vi "FipsAdjacent.vi"() -> (11 "Fips":i32[](array[numeric]))   [LabVIEW 2017] (continued)
WA\"\t53075\t\"Nez Perce County, ID\"\t16069\n\"Whitman County, WA\"\t53075\t\"Adams County, WA\"\t53001\n\"Whitman County, WA\"\t53075\t\"Asotin County, WA\"\t53003\n\"Whitman County, WA\"\t53075\t\"Columbia County, WA\"\t53013\n\"Whitman County, WA\"\t53075\t\"Franklin County, WA\"\t53021\n\"Whitman County, WA\"\t53075\t\"Garfield County, WA\"\t53023\n\"Whitman County, WA\"\t53075\t\"Lincoln County, WA\"\t53043\n\"Whitman County, WA\"\t53075\t\"Spokane County, WA\"\t53063\n\"Whitman County, WA\"\t53075\t\"Whitman County, WA\"\t53075\n\"Yakima County, WA\"\t53077\t\"Benton County, WA\"\t53005\n\"Yakima County, WA\"\t53077\t\"Grant County, WA\"\t53025\n\"Yakima County, WA\"\t53077\t\"King County, WA\"\t53033\n\"Yakima County, WA\"\t53077\t\"Kittitas County, WA\"\t53037\n\"Yakima County, WA\"\t53077\t\"Klickitat County, WA\"\t53039\n\"Yakima County, WA\"\t53077\t\"Lewis County, WA\"\t53041\n\"Yakima County, WA\"\t53077\t\"Pierce County, WA\"\t53053\n\"Yakima County, WA\"\t53077\t\"Skamania County, WA\"\t53059\n\"Yakima County, WA\"\t53077\t\"Yakima County, WA\"\t53077\n\"Barbour County, WV\"\t54001\t\"Barbour County, WV\"\t54001\n\"Barbour County, WV\"\t54001\t\"Harrison County, WV\"\t54033\n\"Barbour County, WV\"\t54001\t\"Preston County, WV\"\t54077\n\"Barbour County, WV\"\t54001\t\"Randolph County, WV\"\t54083\n\"Barbour County, WV\"\t54001\t\"Taylor County, WV\"\t54091\n\"Barbour County, WV\"\t54001\t\"Tucker County, WV\"\t54093\n\"Barbour County, WV\"\t54001\t\"Upshur County, WV\"\t54097\n\"Berkeley County, WV\"\t54003\t\"Washington County, MD\"\t24043\n\"Berkeley County, WV\"\t54003\t\"Clarke County, VA\"\t51043\n\"Berkeley County, WV\"\t54003\t\"Frederick County, VA\"\t51069\n\"Berkeley County, WV\"\t54003\t\"Berkeley County, WV\"\t54003\n\"Berkeley County, WV\"\t54003\t\"Jefferson County, WV\"\t54037\n\"Berkeley County, WV\"\t54003\t\"Morgan County, WV\"\t54065\n\"Boone County, WV\"\t54005\t\"Boone County, WV\"\t54005\n\"Boone County, WV\"\t54005\t\"Kanawha County, WV\"\t54039\n\"Boone County, WV\"\t54005\t\"Lincoln County, WV\"\t54043\n\"Boone County, WV\"\t54005\t\"Logan County, WV\"\t54045\n\"Boone County, WV\"\t54005\t\"Raleigh County, WV\"\t54081\n\"Boone County, WV\"\t54005\t\"Wyoming County, WV\"\t54109\n\"Braxton County, WV\"\t54007\t\"Braxton County, WV\"\t54007\n\"Braxton County, WV\"\t54007\t\"Calhoun County, WV\"\t54013\n\"Braxton County, WV\"\t54007\t\"Clay County, WV\"\t54015\n\"Braxton County, WV\"\t54007\t\"Gilmer County, WV\"\t54021\n\"Braxton County, WV\"\t54007\t\"Lewis County, WV\"\t54041\n\"Braxton County, WV\"\t54007\t\"Nicholas County, WV\"\t54067\n\"Braxton County, WV\"\t54007\t\"Webster County, WV\"\t54101\n\"Brooke County, WV\"\t54009\t\"Jefferson County, OH\"\t39081\n\"Brooke County, WV\"\t54009\t\"Washington County, PA\"\t42125\n\"Brooke County, WV\"\t54009\t\"Brooke County, WV\"\t54009\n\"Brooke County, WV\"\t54009\t\"Hancock County, WV\"\t54029\n\"Brooke County, WV\"\t54009\t\"Ohio County, WV\"\t54069\n\"Cabell County, WV\"\t54011\t\"Gallia County, OH\"\t39053\n\"Cabell County, WV\"\t54011\t\"Lawrence County, OH\"\t39087\n\"Cabell County, WV\"\t54011\t\"Cabell County, WV\"\t54011\n\"Cabell County, WV\"\t54011\t\"Lincoln County, WV\"\t54043\n\"Cabell County, WV\"\t54011\t\"Mason County, WV\"\t54053\n\"Cabell County, WV\"\t54011\t\"Putnam County, WV\"\t54079\n\"Cabell County, WV\"\t54011\t\"Wayne County, WV\"\t54099\n\"Calhoun County, WV\"\t54013\t\"Braxton County, WV\"\t54007\n\"Calhoun County, WV\"\t54013\t\"Calhoun County, WV\"\t54013\n\"Calhoun County, WV\"\t54013\t\"Clay County, WV\"\t54015\n\"Calhoun County, WV\"\t54013\t\"Gilmer County, WV\"\t54021\n\"Calhoun County, WV\"\t54013\t\"Ritchie County, WV\"\t54085\n\"Calhoun County, WV\"\t54013\t\"Roane County, WV\"\t54087\n\"Calhoun County, WV\"\t54013\t\"Wirt County, WV\"\t54105\n\"Clay County, WV\"\t54015\t\"Braxton County, WV\"\t54007\n\"Clay County, WV\"\t54015\t\"Calhoun County, WV\"\t54013\n\"Clay County, WV\"\t54015\t\"Clay County, WV\"\t54015\n\"Clay County, WV\"\t54015\t\"Kanawha County, WV\"\t54039\n\"Clay County, WV\"\t54015\t\"Nicholas County, WV\"\t54067\n\"Clay County, WV\"\t54015\t\"Roane County, WV\"\t54087\n\"Doddridge County, WV\"\t54017\t\"Doddridge County, WV\"\t54017\n\"Doddridge County, WV\"\t54017\t\"Gilmer County, WV\"\t54021\n\"Doddridge County, WV\"\t54017\t\"Harrison County, WV\"\t54033\n\"Doddridge County, WV\"\t54017\t\"Lewis County, WV\"\t54041\n\"Doddridge County, WV\"\t54017\t\"Ritchie County, WV\"\t54085\n\"Doddridge County, WV\"\t54017\t\"Tyler County, WV\"\t54095\n\"Doddridge County, WV\"\t54017\t\"Wetzel County, WV\"\t54103\n\"Fayette County, WV\"\t54019\t\"Fayette County, WV\"\t54019\n\"Fayette County, WV\"\t54019\t\"Greenbrier County, WV\"\t54025\n\"Fayette County, WV\"\t54019\t\"Kanawha County, WV\"\t54039\n\"Fayette County, WV\"\t54019\t\"Nicholas County, WV\"\t54067\n\"Fayette County, WV\"\t54019\t\"Raleigh County, WV\"\t54081\n\"Fayette County, WV\"\t54019\t\"Summers County, WV\"\t54089\n\"Gilmer County, WV\"\t54021\t\"Braxton County, WV\"\t54007\n\"Gilmer County, WV\"\t54021\t\"Calhoun County, WV\"\t54013\n\"Gilmer County, WV\"\t54021\t\"Doddridge County, WV\"\t54017\n\"Gilmer County, WV\"\t54021\t\"Gilmer County, WV\"\t54021\n\"Gilmer County, WV\"\t54021\t\"Lewis County, WV\"\t54041\n\"Gilmer County, WV\"\t54021\t\"Ritchie County, WV\"\t54085\n\"Grant County, WV\"\t54023\t\"Garrett County, MD\"\t24023\n\"Grant County, WV\"\t54023\t\"Grant County, WV\"\t54023\n\"Grant County, WV\"\t54023\t\"Hampshire County, WV\"\t54027\n\"Grant County, WV\"\t54023\t\"Hardy County, WV\"\t54031\n\"Grant County, WV\"\t54023\t\"Mineral County, WV\"\t54057\n\"Grant County, WV\"\t54023\t\"Pendleton County, WV\"\t54071\n\"Grant County, WV\"\t54023\t\"Preston County, WV\"\t54077\n\"Grant County, WV\"\t54023\t\"Randolph County, WV\"\t54083\n\"Grant County, WV\"\t54023\t\"Tucker County, WV\"\t54093\n\"Greenbrier County, WV\"\t54025\t\"Alleghany County, VA\"\t51005\n\"Greenbrier County, WV\"\t54025\t\"Bath County, VA\"\t51017\n\"Greenbrier County, WV\"\t54025\t\"Fayette County, WV\"\t54019\n\"Greenbrier County, WV\"\t54025\t\"Greenbrier County, WV\"\t54025\n\"Greenbrier County, WV\"\t54025\t\"Monroe County, WV\"\t54063\n\"Greenbrier County, WV\"\t54025\t\"Nicholas County, WV\"\t54067\n\"Greenbrier County, WV\"\t54025\t\"Pocahontas County, WV\"\t54075\n\"Greenbrier County, WV\"\t54025\t\"Summers County, WV\"\t54089\n\"Greenbrier County, WV\"\t54025\t\"Webster County, WV\"\t54101\n\"Hampshire County, WV\"\t54027\t\"Allegany County, MD\"\t24001\n\"Hampshire County, WV\"\t54027\t\"Frederick County, VA\"\t51069\n\"Hampshire County, WV\"\t54027\t\"Grant County, WV\"\t54023\n\"Hampshire County, WV\"\t54027\t\"Hampshire County, WV\"\t54027\n\"Hampshire County, WV\"\t54027\t\"Hardy County, WV\"\t54031\n\"Hampshire County, WV\"\t54027\t\"Mineral County, WV\"\t54057\n\"Hampshire County, WV\"\t54027\t\"Morgan County, WV\"\t54065\n\"Hancock County, WV\"\t54029\t\"Columbiana County, OH\"\t39029\n\"Hancock County, WV\"\t54029\t\"Jefferson County, OH\"\t39081\n\"Hancock County, WV\"\t54029\t\"Beaver County, PA\"\t42007\n\"Hancock County, WV\"\t54029\t\"Washington County, PA\"\t42125\n\"Hancock County, WV\"\t54029\t\"Brooke County, WV\"\t54009\n\"Hancock County, WV\"\t54029\t\"Hancock County, WV\"\t54029\n\"Hardy County, WV\"\t54031\t\"Frederick County, VA\"\t51069\n\"Hardy County, WV\"\t54031\t\"Rockingham County, VA\"\t51165\n\"Hardy County, WV\"\t54031\t\"Shenandoah County, VA\"\t51171\n\"Hardy County, WV\"\t54031\t\"Grant County, WV\"\t54023\n\"Hardy County, WV\"\t54031\t\"Hampshire County, WV\"\t54027\n\"Hardy County, WV\"\t54031\t\"Hardy County, WV\"\t54031\n\"Hardy County, WV\"\t54031\t\"Mineral County, WV\"\t54057\n\"Hardy County, WV\"\t54031\t\"Pendleton County, WV\"\t54071\n\"Harrison County, WV\"\t54033\t\"Barbour County, WV\"\t54001\n\"Harrison County, WV\"\t54033\t\"Doddridge County, WV\"\t54017\n\"Harrison County, WV\"\t54033\t\"Harrison County, WV\"\t54033\n\"Harrison County, WV\"\t54033\t\"Lewis County, WV\"\t54041\n\"Harrison County, WV\"\t54033\t\"Marion County, WV\"\t54049\n\"Harrison County, WV\"\t54033\t\"Taylor County, WV\"\t54091\n\"Harrison County, WV\"\t54033\t\"Upshur County, WV\"\t54097\n\"Harrison County, WV\"\t54033\t\"Wetzel County, WV\"\t54103\n\"Jackson County, WV\"\t54035\t\"Meigs County, OH\"\t39105\n\"Jackson County, WV\"\t54035\t\"Jackson County, WV\"\t54035\n\"Jackson County, WV\"\t54035\t\"Kanawha County, WV\"\t54039\n\"Jackson County, WV\"\t54035\t\"Mason County, WV\"\t54053\n\"Jackson County, WV\"\t54035\t\"Putnam County, WV\"\t54079\n\"Jackson County, WV\"\t54035\t\"Roane County, WV\"\t54087\n\"Jackson County, WV\"\t54035\t\"Wirt County, WV\"\t54105\n\"Jackson County, WV\"\t54035\t\"Wood County, WV\"\t54107\n\"Jefferson County, WV\"\t54037\t\"Washington County, MD\"\t24043\n\"Jefferson County, WV\"\t54037\t\"Clarke County, VA\"\t51043\n\"Jefferson County, WV\"\t54037\t\"Frederick County, VA\"\t51069\n\"Jefferson County, WV\"\t54037\t\"Loudoun County, VA\"\t51107\n\"Jefferson County, WV\"\t54037\t\"Berkeley County, WV\"\t54003\n\"Jefferson County, WV\"\t54037\t\"Jefferson County, WV\"\t54037\n\"Kanawha County, WV\"\t54039\t\"Boone County, WV\"\t54005\n\"Kanawha County, WV\"\t54039\t\"Clay County, WV\"\t54015\n\"Kanawha County, WV\"\t54039\t\"Fayette County, WV\"\t54019\n\"Kanawha County, WV\"\t54039\t\"Jackson County, WV\"\t54035\n\"Kanawha County, WV\"\t54039\t\"Kanawha County, WV\"\t54039\n\"Kanawha County, WV\"\t54039\t\"Lincoln County, WV\"\t54043\n\"Kanawha County, WV\"\t54039\t\"Nicholas County, WV\"\t54067\n\"Kanawha County, WV\"\t54039\t\"Putnam County, WV\"\t54079\n\"Kanawha County, WV\"\t54039\t\"Raleigh County, WV\"\t54081\n\"Kanawha County, WV\"\t54039\t\"Roane County, WV\"\t54087\n\"Lewis County, WV\"\t54041\t\"Braxton County, WV\"\t54007\n\"Lewis County, WV\"\t54041\t\"Doddridge County, WV\"\t54017\n\"Lewis County, WV\"\t54041\t\"Gilmer County, WV\"\t54021\n\"Lewis County, WV\"\t54041\t\"Harrison County, WV\"\t54033\n\"Lewis County, WV\"\t54041\t\"Lewis County, WV\"\t54041\n\"Lewis County, WV\"\t54041\t\"Upshur County, WV\"\t54097\n\"Lewis County, WV\"\t54041\t\"Webster County, WV\"\t54101\n\"Lincoln County, WV\"\t54043\t\"Boone County, WV\"\t54005\n\"Lincoln County, WV\"\t54043\t\"Cabell County, WV\"\t54011\n\"Lincoln County, WV\"\t54043\t\"Kanawha County, WV\"\t54039\n\"Lincoln County, WV\"\t54043\t\"Lincoln County, WV\"\t54043\n\"Lincoln County, WV\"\t54043\t\"Logan County, WV\"\t54045\n\"Lincoln County, WV\"\t54043\t\"Mingo County, WV\"\t54059\n\"Lincoln County, WV\"\t54043\t\"Putnam County, WV\"\t54079\n\"Lincoln County, WV\"\t54043\t\"Wayne County, WV\"\t54099\n\"Logan County, WV\"\t54045\t\"Boone County, WV\"\t54005\n\"Logan County, WV\"\t54045\t\"Lincoln County, WV\"\t54043\n\"Logan County, WV\"\t54045\t\"Logan County, WV\"\t54045\n\"Logan County, WV\"\t54045\t\"Mingo County, WV\"\t54059\n\"Logan County, WV\"\t54045\t\"Wyoming County, WV\"\t54109\n\"McDowell County, WV\"\t54047\t\"Buchanan County, VA\"\t51027\n\"McDowell County, WV\"\t54047\t\"Tazewell County, VA\"\t51185\n\"McDowell County, WV\"\t54047\t\"McDowell County, WV\"\t54047\n\"McDowell County, WV\"\t54047\t\"Mercer County, WV\"\t54055\n\"McDowell County, WV\"\t54047\t\"Mingo County, WV\"\t54059\n\"McDowell County, WV\"\t54047\t\"Wyoming County, WV\"\t54109\n\"Marion County, WV\"\t54049\t\"Harrison County, WV\"\t54033\n\"Marion County, WV\"\t54049\t\"Marion County, WV\"\t54049\n\"Marion County, WV\"\t54049\t\"Monongalia County, WV\"\t54061\n\"Marion County, WV\"\t54049\t\"Taylor County, WV\"\t54091\n\"Marion County, WV\"\t54049\t\"Wetzel County, WV\"\t54103\n\"Marshall County, WV\"\t54051\t\"Belmont County, OH\"\t39013\n\"Marshall County, WV\"\t54051\t\"Monroe County, OH\"\t39111\n\"Marshall County, WV\"\t54051\t\"Greene County, PA\"\t42059\n\"Marshall County, WV\"\t54051\t\"Washington County, PA\"\t42125\n\"Marshall County, WV\"\t54051\t\"Marshall County, WV\"\t54051\n\"Marshall County, WV\"\t54051\t\"Ohio County, WV\"\t54069\n\"Marshall County, WV\"\t54051\t\"Wetzel County, WV\"\t54103\n\"Mason County, WV\"\t54053\t\"Gallia County, OH\"\t39053\n\"Mason County, WV\"\t54053\t\"Meigs County, OH\"\t39105\n\"Mason County, WV\"\t54053\t\"Cabell County, WV\"\t54011\n\"Mason County, WV\"\t54053\t\"Jackson County, WV\"\t54035\n\"Mason County, WV\"\t54053\t\"Mason County, WV\"\t54053\n\"Mason County, WV\"\t54053\t\"Putnam County, WV\"\t54079\n\"Mercer County, WV\"\t54055\t\"Bland County, VA\"\t51021\n\"Mercer County, WV\"\t54055\t\"Giles County, VA\"\t51071\n\"Mercer County, WV\"\t54055\t\"Tazewell County, VA\"\t51185\n\"Mercer County, WV\"\t54055\t\"McDowell County, WV\"\t54047\n\"Mercer County, WV\"\t54055\t\"Mercer County, WV\"\t54055\n\"Mercer County, WV\"\t54055\t\"Raleigh County, WV\"\t54081\n\"Mercer County, WV\"\t54055\t\"Summers County, WV\"\t54089\n\"Mercer County, WV\"\t54055\t\"Wyoming County, WV\"\t54109\n\"Mineral County, WV\"\t54057\t\"Allegany County, MD\"\t24001\n\"Mineral County, WV\"\t54057\t\"Garrett County, MD\"\t24023\n\"Mineral County, WV\"\t54057\t\"Grant County, WV\"\t54023\n\"Mineral County, WV\"\t54057\t\"Hampshire County, WV\"\t54027\n\"Mineral County, WV\"\t54057\t\"Hardy County, WV\"\t54031\n\"Mineral County, WV\"\t54057\t\"Mineral County, WV\"\t54057\n\"Mingo County, WV\"\t54059\t\"Martin County, KY\"\t21159\n\"Mingo County, WV\"\t54059\t\"Pike County, KY\"\t21195\n\"Mingo County, WV\"\t54059\t\"Buchanan County, VA\"\t51027\n\"Mingo County, WV\"\t54059\t\"Lincoln County, WV\"\t54043\n\"Mingo County, WV\"\t54059\t\"Logan County, WV\"\t54045\n\"Mingo County, WV\"\t54059\t\"McDowell County, WV\"\t54047\n\"Mingo County, WV\"\t54059\t\"Mingo County, WV\"\t54059\n\"Mingo County, WV\"\t54059\t\"Wayne County, WV\"\t54099\n\"Mingo County, WV\"\t54059\t\"Wyoming County, WV\"\t54109\n\"Monongalia County, WV\"\t54061\t\"Fayette County, PA\"\t42051\n\"Monongalia County, WV\"\t54061\t\"Greene County, PA\"\t42059\n\"Monongalia County, WV\"\t54061\t\"Marion County, WV\"\t54049\n\"Monongalia County, WV\"\t54061\t\"Monongalia County, WV\"\t54061\n\"Monongalia County, WV\"\t54061\t\"Preston County, WV\"\t54077\n\"Monongalia County, WV\"\t54061\t\"Taylor County, WV\"\t54091\n\"Monongalia County, WV\"\t54061\t\"Wetzel County, WV\"\t54103\n\"Monroe County, WV\"\t54063\t\"Alleghany County, VA\"\t51005\n\"Monroe County, WV\"\t54063\t\"Craig County, VA\"\t51045\n\"Monroe County, WV\"\t54063\t\"Giles County, VA\"\t51071\n\"Monroe County, WV\"\t54063\t\"Greenbrier County, WV\"\t54025\n\"Monroe County, WV\"\t54063\t\"Monroe County, WV\"\t54063\n\"Monroe County, WV\"\t54063\t\"Summers County, WV\"\t54089\n\"Morgan County, WV\"\t54065\t\"Allegany County, MD\"\t24001\n\"Morgan County, WV\"\t54065\t\"Washington County, MD\"\t24043\n\"Morgan County, WV\"\t54065\t\"Frederick County, VA\"\t51069\n\"Morgan County, WV\"\t54065\t\"Berkeley County, WV\"\t54003\n\"Morgan County, WV\"\t54065\t\"Hampshire County, WV\"\t54027\n\"Morgan County, WV\"\t54065\t\"Morgan County, WV\"\t54065\n\"Nicholas County, WV\"\t54067\t\"Braxton County, WV\"\t54007\n\"Nicholas County, WV\"\t54067\t\"Clay County, WV\"\t54015\n\"Nicholas County, WV\"\t54067\t\"Fayette County, WV\"\t54019\n\"Nicholas County, WV\"\t54067\t\"Greenbrier County, WV\"\t54025\n\"Nicholas County, WV\"\t54067\t\"Kanawha County, WV\"\t54039\n\"Nicholas County, WV\"\t54067\t\"Nicholas County, WV\"\t54067\n\"Nicholas County, WV\"\t54067\t\"Webster County, WV\"\t54101\n\"Ohio County, WV\"\t54069\t\"Belmont County, OH\"\t39013\n\"Ohio County, WV\"\t54069\t\"Jefferson County, OH\"\t39081\n\"Ohio County, WV\"\t54069\t\"Washington County, PA\"\t42125\n\"Ohio County, WV\"\t54069\t\"Brooke County, WV\"\t54009\n\"Ohio County, WV\"\t54069\t\"Marshall County, WV\"\t54051\n\"Ohio County, WV\"\t54069\t\"Ohio County, WV\"\t54069\n\"Pendleton County, WV\"\t54071\t\"Augusta County, VA\"\t51015\n\"Pendleton County, WV\"\t54071\t\"Highland County, VA\"\t51091\n\"Pendleton County, WV\"\t54071\t\"Rockingham County, VA\"\t51165\n\"Pendleton County, WV\"\t54071\t\"Grant County, WV\"\t54023\n\"Pendleton County, WV\"\t54071\t\"Hardy County, WV\"\t54031\n\"Pendleton County, WV\"\t54071\t\"Pendleton County, WV\"\t54071\n\"Pendleton County, WV\"\t54071\t\"Pocahontas County, WV\"\t54075\n\"Pendleton County, WV\"\t54071\t\"Randolph County, WV\"\t54083\n\"Pleasants County, WV\"\t54073\t\"Washington County, OH\"\t39167\n\"Pleasants County, WV\"\t54073\t\"Pleasants County, WV\"\t54073\n\"Pleasants County, WV\"\t54073\t\"Ritchie County, WV\"\t54085\n\"Pleasants County, WV\"\t54073\t\"Tyler County, WV\"\t54095\n\"Pleasants County, WV\"\t54073\t\"Wood County, WV\"\t54107\n\"Pocahontas County, WV\"\t54075\t\"Bath County, VA\"\t51017\n\"Pocahontas County, WV\"\t54075\t\"Highland County, VA\"\t51091\n\"Pocahontas County, WV\"\t54075\t\"Greenbrier County, WV\"\t54025\n\"Pocahontas County, WV\"\t54075\t\"Pendleton County, WV\"\t54071\n\"Pocahontas County, WV\"\t54075\t\"Pocahontas County, WV\"\t54075\n\"Pocahontas County, WV\"\t54075\t\"Randolph County, WV\"\t54083\n\"Pocahontas County, WV\"\t54075\t\"Webster County, WV\"\t54101\n\"Preston County, WV\"\t54077\t\"Garrett County, MD\"\t24023\n\"Preston County, WV\"\t54077\t\"Fayette County, PA\"\t42051\n\"Preston County, WV\"\t54077\t\"Barbour County, WV\"\t54001\n\"Preston County, WV\"\t54077\t\"Grant County, WV\"\t54023\n\"Preston County, WV\"\t54077\t\"Monongalia County, WV\"\t54061\n\"Preston County, WV\"\t54077\t\"Preston County, WV\"\t54077\n\"Preston County, WV\"\t54077\t\"Taylor County, WV\"\t54091\n\"Preston County, WV\"\t54077\t\"Tucker County, WV\"\t54093\n\"Putnam County, WV\"\t54079\t\"Cabell County, WV\"\t54011\n\"Putnam County, WV\"\t54079\t\"Jackson County, WV\"\t54035\n\"Putnam County, WV\"\t54079\t\"Kanawha County, WV\"\t54039\n\"Putnam County, WV\"\t54079\t\"Lincoln County, WV\"\t54043\n\"Putnam County, WV\"\t54079\t\"Mason County, WV\"\t54053\n\"Putnam County, WV\"\t54079\t\"Putnam County, WV\"\t54079\n\"Raleigh County, WV\"\t54081\t\"Boone County, WV\"\t54005\n\"Raleigh County, WV\"\t54081\t\"Fayette County, WV\"\t54019\n\"Raleigh County, WV\"\t54081\t\"Kanawha County, WV\"\t54039\n\"Raleigh County, WV\"\t54081\t\"Mercer County, WV\"\t54055\n\"Raleigh County, WV\"\t54081\t\"Raleigh County, WV\"\t54081\n\"Raleigh County, WV\"\t54081\t\"Summers County, WV\"\t54089\n\"Raleigh County, WV\"\t54081\t\"Wyoming County, WV\"\t54109\n\"Randolph County, WV\"\t54083\t\"Barbour County, WV\"\t54001\n\"Randolph County, WV\"\t54083\t\"Grant County, WV\"\t54023\n\"Randolph County, WV\"\t54083\t\"Pendleton County, WV\"\t54071\n\"Randolph County, WV\"\t54083\t\"Pocahontas County, WV\"\t54075\n\"Randolph County, WV\"\t54083\t\"Randolph County, WV\"\t54083\n\"Randolph County, WV\"\t54083\t\"Tucker County, WV\"\t54093\n\"Randolph County, WV\"\t54083\t\"Upshur County, WV\"\t54097\n\"Randolph County, WV\"\t54083\t\"Webster County, WV\"\t54101\n\"Ritchie County, WV\"\t54085\t\"Calhoun County, WV\"\t54013\n\"Ritchie County, WV\"\t54085\t\"Doddridge County, WV\"\t54017\n\"Ritchie County, WV\"\t54085\t\"Gilmer County, WV\"\t54021\n\"Ritchie County, WV\"\t54085\t\"Pleasants County, WV\"\t54073\n\"Ritchie County, WV\"\t54085\t\"Ritchie County, WV\"\t54085\n\"Ritchie County, WV\"\t54085\t\"Tyler County, WV\"\t54095\n\"Ritchie County, WV\"\t54085\t\"Wirt County, WV\"\t54105\n\"Ritchie County, WV\"\t54085\t\"Wood County, WV\"\t54107\n\"Roane County, WV\"\t54087\t\"Calhoun County, WV\"\t54013\n\"Roane County, WV\"\t54087\t\"Clay County, WV\"\t54015\n\"Roane County, WV\"\t54087\t\"Jackson County, WV\"\t54035\n\"Roane County, WV\"\t54087\t\"Kanawha County, WV\"\t54039\n\"Roane County, WV\"\t54087\t\"Roane County, WV\"\t54087\n\"Roane County, WV\"\t54087\t\"Wirt County, WV\"\t54105\n\"Summers County, WV\"\t54089\t\"Giles County, VA\"\t51071\n\"Summers County, WV\"\t54089\t\"Fayette County, WV\"\t54019\n\"Summers County, WV\"\t54089\t\"Greenbrier County, WV\"\t54025\n\"Summers County, WV\"\t54089\t\"Mercer County, WV\"\t54055\n\"Summers County, WV\"\t54089\t\"Monroe County, WV\"\t54063\n\"Summers County, WV\"\t54089\t\"Raleigh County, WV\"\t54081\n\"Summers County, WV\"\t54089\t\"Summers County, WV\"\t54089\n\"Taylor County, WV\"\t54091\t\"Barbour County, WV\"\t54001\n\"Taylor County, WV\"\t54091\t\"Harrison County, WV\"\t54033\n\"Taylor County, WV\"\t54091\t\"Marion County, WV\"\t54049\n\"Taylor County, WV\"\t54091\t\"Monongalia County, WV\"\t54061\n\"Taylor County, WV\"\t54091\t\"Preston County, WV\"\t54077\n\"Taylor County, WV\"\t54091\t\"Taylor County, WV\"\t54091\n\"Tucker County, WV\"\t54093\t\"Barbour County, WV\"\t54001\n\"Tucker County, WV\"\t54093\t\"Grant County, WV\"\t54023\n\"Tucker County, WV\"\t54093\t\"Preston County, WV\"\t54077\n\"Tucker County, WV\"\t54093\t\"Randolph County, WV\"\t54083\n\"Tucker County, WV\"\t54093\t\"Tucker County, WV\"\t54093\n\"Tyler County, WV\"\t54095\t\"Monroe County, OH\"\t39111\n\"Tyler County, WV\"\t54095\t\"Washington County, OH\"\t39167\n\"Tyler County, WV\"\t54095\t\"Doddridge County, WV\"\t54017\n\"Tyler County, WV\"\t54095\t\"Pleasants County, WV\"\t54073\n\"Tyler County, WV\"\t54095\t\"Ritchie County, WV\"\t54085\n\"Tyler County, WV\"\t54095\t\"Tyler County, WV\"\t54095\n\"Tyler County, WV\"\t54095\t\"Wetzel County, WV\"\t54103\n\"Upshur County, WV\"\t54097\t\"Barbour County, WV\"\t54001\n\"Upshur County, WV\"\t54097\t\"Harrison County, WV\"\t54033\n\"Upshur County, WV\"\t54097\t\"Lewis County, WV\"\t54041\n\"Upshur County, WV\"\t54097\t\"Randolph County, WV\"\t54083\n\"Upshur County, WV\"\t54097\t\"Upshur County, WV\"\t54097\n\"Upshur County, WV\"\t54097\t\"Webster County, WV\"\t54101\n\"Wayne County, WV\"\t54099\t\"Boyd County, KY\"\t21019\n\"Wayne County, WV\"\t54099\t\"Lawrence County, KY\"\t21127\n\"Wayne County, WV\"\t54099\t\"Martin County, KY\"\t21159\n\"Wayne County, WV\"\t54099\t\"Lawrence County, OH\"\t39087\n\"Wayne County, WV\"\t54099\t\"Cabell County, WV\"\t54011\n\"Wayne County, WV\"\t54099\t\"Lincoln County, WV\"\t54043\n\"Wayne County, WV\"\t54099\t\"Mingo County, WV\"\t54059\n\"Wayne County, WV\"\t54099\t\"Wayne County, WV\"\t54099\n\"Webster County, WV\"\t54101\t\"Braxton County, WV\"\t54007\n\"Webster County, WV\"\t54101\t\"Greenbrier County, WV\"\t54025\n\"Webster County, WV\"\t54101\t\"Lewis County, WV\"\t54041\n\"Webster County, WV\"\t54101\t\"Nicholas County, WV\"\t54067\n\"Webster County, WV\"\t54101\t\"Pocahontas County, WV\"\t54075\n\"Webster County, WV\"\t54101\t\"Randolph County, WV\"\t54083\n\"Webster County, WV\"\t54101\t\"Upshur County, WV\"\t54097\n\"Webster County, WV\"\t54101\t\"Webster County, WV\"\t54101\n\"Wetzel County, WV\"\t54103\t\"Monroe County, OH\"\t39111\n\"Wetzel County, WV\"\t54103\t\"Greene County, PA\"\t42059\n\"Wetzel County, WV\"\t54103\t\"Doddridge County, WV\"\t54017\n\"Wetzel County, WV\"\t54103\t\"Harrison County, WV\"\t54033\n\"Wetzel County, WV\"\t54103\t\"Marion County, WV\"\t54049\n\"Wetzel County, WV\"\t54103\t\"Marshall County, WV\"\t54051\n\"Wetzel County, WV\"\t54103\t\"Monongalia County, WV\"\t54061\n\"Wetzel County, WV\"\t54103\t\"Tyler County, WV\"\t54095\n\"Wetzel County, WV\"\t54103\t\"Wetzel County, WV\"\t54103\n\"Wirt County, WV\"\t54105\t\"Calhoun County, WV\"\t54013\n\"Wirt County, WV\"\t54105\t\"Jackson County, WV\"\t54035\n\"Wirt County, WV\"\t54105\t\"Ritchie County, WV\"\t54085\n\"Wirt County, WV\"\t54105\t\"Roane County, WV\"\t54087\n\"Wirt County, WV\"\t54105\t\"Wirt County, WV\"\t54105\n\"Wirt County, WV\"\t54105\t\"Wood County, WV\"\t54107\n\"Wood County, WV\"\t54107\t\"Athens County, OH\"\t39009\n\"Wood County, WV\"\t54107\t\"Meigs County, OH\"\t39105\n\"Wood County, WV\"\t54107\t\"Washington County, OH\"\t39167\n\"Wood County, WV\"\t54107\t\"Jackson County, WV\"\t54035\n\"Wood County, WV\"\t54107\t\"Pleasants County, WV\"\t54073\n\"Wood County, WV\"\t54107\t\"Ritchie County, WV\"\t54085\n\"Wood County, WV\"\t54107\t\"Wirt County, WV\"\t54105\n\"Wood County, WV\"\t54107\t\"Wood County, WV\"\t54107\n\"Wyoming County, WV\"\t54109\t\"Boone County, WV\"\t54005\n\"Wyoming County, WV\"\t54109\t\"Logan County, WV\"\t54045\n\"Wyoming County, WV\"\t54109\t\"McDowell County, WV\"\t54047\n\"Wyoming County, WV\"\t54109\t\"Mercer County, WV\"\t54055\n\"Wyoming County, WV\"\t54109\t\"Mingo County, WV\"\t54059\n\"Wyoming County, WV\"\t54109\t\"Raleigh County, WV\"\t54081\n\"Wyoming County, WV\"\t54109\t\"Wyoming County, WV\"\t54109\n\"Adams County, WI\"\t55001\t\"Adams County, WI\"\t55001\n\"Adams County, WI\"\t55001\t\"Columbia County, WI\"\t55021\n\"Adams County, WI\"\t55001\t\"Juneau County, WI\"\t55057\n\"Adams County, WI\"\t55001\t\"Marquette County, WI\"\t55077\n\"Adams County, WI\"\t55001\t\"Portage County, WI\"\t55097\n\"Adams County, WI\"\t55001\t\"Sauk County, WI\"\t55111\n\"Adams County, WI\"\t55001\t\"Waushara County, WI\"\t55137\n\"Adams County, WI\"\t55001\t\"Wood County, WI\"\t55141\n\"Ashland County, WI\"\t55003\t\"Gogebic County, MI\"\t26053\n\"Ashland County, WI\"\t55003\t\"Ontonagon County, MI\"\t26131\n\"Ashland County, WI\"\t55003\t\"Cook County, MN\"\t27031\n\"Ashland County, WI\"\t55003\t\"Lake County, MN\"\t27075\n\"Ashland County, WI\"\t55003\t\"Ashland County, WI\"\t55003\n\"Ashland County, WI\"\t55003\t\"Bayfield County, WI\"\t55007\n\"Ashland County, WI\"\t55003\t\"Iron County, WI\"\t55051\n\"Ashland County, WI\"\t55003\t\"Price County, WI\"\t55099\n\"Ashland County, WI\"\t55003\t\"Sawyer County, WI\"\t55113\n\"Barron County, WI\"\t55005\t\"Barron County, WI\"\t55005\n\"Barron County, WI\"\t55005\t\"Burnett County, WI\"\t55013\n\"Barron County, WI\"\t55005\t\"Chippewa County, WI\"\t55017\n\"Barron County, WI\"\t55005\t\"Dunn County, WI\"\t55033\n\"Barron County, WI\"\t55005\t\"Polk County, WI\"\t55095\n\"Barron County, WI\"\t55005\t\"Rusk County, WI\"\t55107\n\"Barron County, WI\"\t55005\t\"St. Croix County, WI\"\t55109\n\"Barron County, WI\"\t55005\t\"Sawyer County, WI\"\t55113\n\"Barron County, WI\"\t55005\t\"Washburn County, WI\"\t55129\n\"Bayfield County, WI\"\t55007\t\"Lake County, MN\"\t27075\n\"Bayfield County, WI\"\t55007\t\"Ashland County, WI\"\t55003\n\"Bayfield County, WI\"\t55007\t\"Bayfield County, WI\"\t55007\n\"Bayfield County, WI\"\t55007\t\"Douglas County, WI\"\t55031\n\"Bayfield County, WI\"\t55007\t\"Sawyer County, WI\"\t55113\n\"Bayfield County, WI\"\t55007\t\"Washburn County, WI\"\t55129\n\"Brown County, WI\"\t55009\t\"Brown County, WI\"\t55009\n\"Brown County, WI\"\t55009\t\"Calumet County, WI\"\t55015\n\"Brown County, WI\"\t55009\t\"Door County, WI\"\t55029\n\"Brown County, WI\"\t55009\t\"Kewaunee County, WI\"\t55061\n\"Brown County, WI\"\t55009\t\"Manitowoc County, WI\"\t55071\n\"Brown County, WI\"\t55009\t\"Oconto County, WI\"\t55083\n\"Brown County, WI\"\t55009\t\"Outagamie County, WI\"\t55087\n\"Brown County, WI\"\t55009\t\"Shawano County, WI\"\t55115\n\"Buffalo County, WI\"\t55011\t\"Wabasha County, MN\"\t27157\n\"Buffalo County, WI\"\t55011\t\"Winona County, MN\"\t27169\n\"Buffalo County, WI\"\t55011\t\"Buffalo County, WI\"\t55011\n\"Buffalo County, WI\"\t55011\t\"Eau Claire County, WI\"\t55035\n\"Buffalo County, WI\"\t55011\t\"Pepin County, WI\"\t55091\n\"Buffalo County, WI\"\t55011\t\"Trempealeau County, WI\"\t55121\n\"Burnett County, WI\"\t55013\t\"Chisago County, MN\"\t27025\n\"Burnett County, WI\"\t55013\t\"Pine County, MN\"\t27115\n\"Burnett County, WI\"\t55013\t\"Barron County, WI\"\t55005\n\"Burnett County, WI\"\t55013\t\"Burnett County, WI\"\t55013\n\"Burnett County, WI\"\t55013\t\"Douglas County, WI\"\t55031\n\"Burnett County, WI\"\t55013\t\"Polk County, WI\"\t55095\n\"Burnett County, WI\"\t55013\t\"Washburn County, WI\"\t55129\n\"Calumet County, WI\"\t55015\t\"Brown County, WI\"\t55009\n\"Calumet County, WI\"\t55015\t\"Calumet County, WI\"\t55015\n\"Calumet County, WI\"\t55015\t\"Fond du Lac County, WI\"\t55039\n\"Calumet County, WI\"\t55015\t\"Manitowoc County, WI\"\t55071\n\"Calumet County, WI\"\t55015\t\"Outagamie County, WI\"\t55087\n\"Calumet County, WI\"\t55015\t\"Sheboygan County, WI\"\t55117\n\"Calumet County, WI\"\t55015\t\"Winnebago County, WI\"\t55139\n\"Chippewa County, WI\"\t55017\t\"Barron County, WI\"\t55005\n\"Chippewa County, WI\"\t55017\t\"Chippewa County, WI\"\t55017\n\"Chippewa County, WI\"\t55017\t\"Clark County, WI\"\t55019\n\"Chippewa County, WI\"\t55017\t\"Dunn County, WI\"\t55033\n\"Chippewa County, WI\"\t55017\t\"Eau Claire County, WI\"\t55035\n\"Chippewa County, WI\"\t55017\t\"Rusk County, WI\"\t55107\n\"Chippewa County, WI\"\t55017\t\"Taylor County, WI\"\t55119\n\"Clark County, WI\"\t55019\t\"Chippewa County, WI\"\t55017\n\"Clark County, WI\"\t55019\t\"Clark County, WI\"\t55019\n\"Clark County, WI\"\t55019\t\"Eau Claire County, WI\"\t55035\n\"Clark County, WI\"\t55019\t\"Jackson County, WI\"\t55053\n\"Clark County, WI\"\t55019\t\"Marathon County, WI\"\t55073\n\"Clark County, WI\"\t55019\t\"Taylor County, WI\"\t55119\n\"Clark County, WI\"\t55019\t\"Wood County, WI\"\t55141\n\"Columbia County, WI\"\t55021\t\"Adams County, WI\"\t55001\n\"Columbia County, WI\"\t55021\t\"Columbia County, WI\"\t55021\n\"Columbia County, WI\"\t55021\t\"Dane County, WI\"\t55025\n\"Columbia County, WI\"\t55021\t\"Dodge County, WI\"\t55027\n\"Columbia County, WI\"\t55021\t\"Green Lake County, WI\"\t55047\n\"Columbia County, WI\"\t55021\t\"Juneau County, WI\"\t55057\n\"Columbia County, WI\"\t55021\t\"Marquette County, WI\"\t55077\n\"Columbia County, WI\"\t55021\t\"Sauk County, WI\"\t55111\n\"Crawford County, WI\"\t55023\t\"Allamakee County, IA\"\t19005\n\"Crawford County, WI\"\t55023\t\"Clayton County, IA\"\t19043\n\"Crawford County, WI\"\t55023\t\"Crawford County, WI\"\t55023\n\"Crawford County, WI\"\t55023\t\"Grant County, WI\"\t55043\n\"Crawford County, WI\"\t55023\t\"Richland County, WI\"\t55103\n\"Crawford County, WI\"\t55023\t\"Vernon County, WI\"\t55123\n\"Dane County, WI\"\t55025\t\"Columbia County, WI\"\t55021\n\"Dane County, WI\"\t55025\t\"Dane County, WI\"\t55025\n\"Dane County, WI\"\t55025\t\"Dodge County, WI\"\t55027\n\"Dane County, WI\"\t55025\t\"Green County, WI\"\t55045\n\"Dane County, WI\"\t55025\t\"Iowa County, WI\"\t55049\n\"Dane County, WI\"\t55025\t\"Jefferson County, WI\"\t55055\n\"Dane County, WI\"\t55025\t\"Rock County, WI\"\t55105\n\"Dane County, WI\"\t55025\t\"Sauk County, WI\"\t55111\n\"Dodge County, WI\"\t55027\t\"Columbia County, WI\"\t55021\n\"Dodge County, WI\"\t55027\t\"Dane County, WI\"\t55025\n\"Dodge County, WI\"\t55027\t\"Dodge County, WI\"\t55027\n\"Dodge County, WI\"\t55027\t\"Fond du Lac County, WI\"\t55039\n\"Dodge County, WI\"\t55027\t\"Green Lake County, WI\"\t55047\n\"Dodge County, WI\"\t55027\t\"Jefferson County, WI\"\t55055\n\"Dodge County, WI\"\t55027\t\"Washington County, WI\"\t55131\n\"Dodge County, WI\"\t55027\t\"Waukesha County, WI\"\t55133\n\"Door County, WI\"\t55029\t\"Benzie County, MI\"\t26019\n\"Door County, WI\"\t55029\t\"Delta County, MI\"\t26041\n\"Door County, WI\"\t55029\t\"Leelanau County, MI\"\t26089\n\"Door County, WI\"\t55029\t\"Menominee County, MI\"\t26109\n\"Door County, WI\"\t55029\t\"Brown County, WI\"\t55009\n\"Door County, WI\"\t55029\t\"Door County, WI\"\t55029\n\"Door County, WI\"\t55029\t\"Kewaunee County, WI\"\t55061\n\"Door County, WI\"\t55029\t\"Marinette County, WI\"\t55075\n\"Door County, WI\"\t55029\t\"Oconto County, WI\"\t55083\n\"Douglas County, WI\"\t55031\t\"Carlton County, MN\"\t27017\n\"Douglas County, WI\"\t55031\t\"Lake County, MN\"\t27075\n\"Douglas County, WI\"\t55031\t\"Pine County, MN\"\t27115\n\"Douglas County, WI\"\t55031\t\"St. Louis County, MN\"\t27137\n\"Douglas County, WI\"\t55031\t\"Bayfield County, WI\"\t55007\n\"Douglas County, WI\"\t55031\t\"Burnett County, WI\"\t55013\n\"Douglas County, WI\"\t55031\t\"Douglas County, WI\"\t55031\n\"Douglas County, WI\"\t55031\t\"Sawyer County, WI\"\t55113\n\"Douglas County, WI\"\t55031\t\"Washburn County, WI\"\t55129\n\"Dunn County, WI\"\t55033\t\"Barron County, WI\"\t55005\n\"Dunn County, WI\"\t55033\t\"Chippewa County, WI\"\t55017\n\"Dunn County, WI\"\t55033\t\"Dunn County, WI\"\t55033\n\"Dunn County, WI\"\t55033\t\"Eau Claire County, WI\"\t55035\n\"Dunn County, WI\"\t55033\t\"Pepin County, WI\"\t55091\n\"Dunn County, WI\"\t55033\t\"Pierce County, WI\"\t55093\n\"Dunn County, WI\"\t55033\t\"Polk County, WI\"\t55095\n\"Dunn County, WI\"\t55033\t\"St. Croix County, WI\"\t55109\n\"Eau Claire County, WI\"\t55035\t\"Buffalo County, WI\"\t55011\n\"Eau Claire County, WI\"\t55035\t\"Chippewa County, WI\"\t55017\n\"Eau Claire County, WI\"\t55035\t\"Clark County, WI\"\t55019\n\"Eau Claire County, WI\"\t55035\t\"Dunn County, WI\"\t55033\n\"Eau Claire County, WI\"\t55035\t\"Eau Claire County, WI\"\t55035\n\"Eau Claire County, WI\"\t55035\t\"Jackson County, WI\"\t55053\n\"Eau Claire County, WI\"\t55035\t\"Pepin County, WI\"\t55091\n\"Eau Claire County, WI\"\t55035\t\"Trempealeau County, WI\"\t55121\n\"Florence County, WI\"\t55037\t\"Dickinson County, MI\"\t26043\n\"Florence County, WI\"\t55037\t\"Iron County, MI\"\t26071\n\"Florence County, WI\"\t55037\t\"Florence County, WI\"\t55037\n\"Florence County, WI\"\t55037\t\"Forest County, WI\"\t55041\n\"Florence County, WI\"\t55037\t\"Marinette County, WI\"\t55075\n\"Fond du Lac County, WI\"\t55039\t\"Calumet County, WI\"\t55015\n\"Fond du Lac County, WI\"\t55039\t\"Dodge County, WI\"\t55027\n\"Fond du Lac County, WI\"\t55039\t\"Fond du Lac County, WI\"\t55039\n\"Fond du Lac County, WI\"\t55039\t\"Green Lake County, WI\"\t55047\n\"Fond du Lac County, WI\"\t55039\t\"Sheboygan County, WI\"\t55117\n\"Fond du Lac County, WI\"\t55039\t\"Washington County, WI\"\t55131\n\"Fond du Lac County, WI\"\t55039\t\"Winnebago County, WI\"\t55139\n\"Forest County, WI\"\t55041\t\"Iron County, MI\"\t26071\n\"Forest County, WI\"\t55041\t\"Florence County, WI\"\t55037\n\"Forest County, WI\"\t55041\t\"Forest County, WI\"\t55041\n\"Forest County, WI\"\t55041\t\"Langlade County, WI\"\t55067\n\"Forest County, WI\"\t55041\t\"Marinette County, WI\"\t55075\n\"Forest County, WI\"\t55041\t\"Oconto County, WI\"\t55083\n\"Forest County, WI\"\t55041\t\"Oneida County, WI\"\t55085\n\"Forest County, WI\"\t55041\t\"Vilas County, WI\"\t55125\n\"Grant County, WI\"\t55043\t\"Jo Daviess County, IL\"\t17085\n\"Grant County, WI\"\t55043\t\"Clayton County, IA\"\t19043\n\"Grant County, WI\"\t55043\t\"Dubuque County, IA\"\t19061\n\"Grant County, WI\"\t55043\t\"Crawford County, WI\"\t55023\n\"Grant County, WI\"\t55043\t\"Grant County, WI\"\t55043\n\"Grant County, WI\"\t55043\t\"Iowa County, WI\"\t55049\n\"Grant County, WI\"\t55043\t\"Lafayette County, WI\"\t55065\n\"Grant County, WI\"\t55043\t\"Richland County, WI\"\t55103\n\"Green County, WI\"\t55045\t\"Stephenson County, IL\"\t17177\n\"Green County, WI\"\t55045\t\"Winnebago County, IL\"\t17201\n\"Green County, WI\"\t55045\t\"Dane County, WI\"\t55025\n\"Green County, WI\"\t55045\t\"Green County, WI\"\t55045\n\"Green County, WI\"\t55045\t\"Iowa County, WI\"\t55049\n\"Green County, WI\"\t55045\t\"Lafayette County, WI\"\t55065\n\"Green County, WI\"\t55045\t\"Rock County, WI\"\t55105\n\"Green Lake County, WI\"\t55047\t\"Columbia County, WI\"\t55021\n\"Green Lake County, WI\"\t55047\t\"Dodge County, WI\"\t55027\n\"Green Lake County, WI\"\t55047\t\"Fond du Lac County, WI\"\t55039\n\"Green Lake County, WI\"\t55047\t\"Green Lake County, WI\"\t55047\n\"Green Lake County, WI\"\t55047\t\"Marquette County, WI\"\t55077\n\"Green Lake County, WI\"\t55047\t\"Waushara County, WI\"\t55137\n\"Green Lake County, WI\"\t55047\t\"Winnebago County, WI\"\t55139\n\"Iowa County, WI\"\t55049\t\"Dane County, WI\"\t55025\n\"Iowa County, WI\"\t55049\t\"Grant County, WI\"\t55043\n\"Iowa County, WI\"\t55049\t\"Green County, WI\"\t55045\n\"Iowa County, WI\"\t55049\t\"Iowa County, WI\"\t55049\n\"Iowa County, WI\"\t55049\t\"Lafayette County, WI\"\t55065\n\"Iowa County, WI\"\t55049\t\"Richland County, WI\"\t55103\n\"Iowa County, WI\"\t55049\t\"Sauk County, WI\"\t55111\n\"Iron County, WI\"\t55051\t\"Gogebic County, MI\"\t26053\n\"Iron County, WI\"\t55051\t\"Ashland County, WI\"\t55003\n\"Iron County, WI\"\t55051\t\"Iron County, WI\"\t55051\n\"Iron County, WI\"\t55051\t\"Price County, WI\"\t55099\n\"Iron County, WI\"\t55051\t\"Vilas County, WI\"\t55125\n\"Jackson County, WI\"\t55053\t\"Clark County, WI\"\t55019\n\"Jackson County, WI\"\t55053\t\"Eau Claire County, WI\"\t55035\n\"Jackson County, WI\"\t55053\t\"Jackson County, WI\"\t55053\n\"Jackson County, WI\"\t55053\t\"Juneau County, WI\"\t55057\n\"Jackson County, WI\"\t55053\t\"La Crosse County, WI\"\t55063\n\"Jackson County, WI\"\t55053\t\"Monroe County, WI\"\t55081\n\"Jackson County, WI\"\t55053\t\"Trempealeau County, WI\"\t55121\n\"Jackson County, WI\"\t55053\t\"Wood County, WI\"\t55141\n\"Jefferson County, WI\"\t55055\t\"Dane County, WI\"\t55025\n\"Jefferson County, WI\"\t55055\t\"Dodge County, WI\"\t55027\n\"Jefferson County, WI\"\t55055\t\"Jefferson County, WI\"\t55055\n\"Jefferson County, WI\"\t55055\t\"Rock County, WI\"\t55105\n\"Jefferson County, WI\"\t55055\t\"Walworth County, WI\"\t55127\n\"Jefferson County, WI\"\t55055\t\"Waukesha County, WI\"\t55133\n\"Juneau County, WI\"\t55057\t\"Adams County, WI\"\t55001\n\"Juneau County, WI\"\t55057\t\"Columbia County, WI\"\t55021\n\"Juneau County, WI\"\t55057\t\"Jackson County, WI\"\t55053\n\"Juneau County, WI\"\t55057\t\"Juneau County, WI\"\t55057\n\"Juneau County, WI\"\t55057\t\"Monroe County, WI\"\t55081\n\"Juneau County, WI\"\t55057\t\"Sauk County, WI\"\t55111\n\"Juneau County, WI\"\t55057\t\"Vernon County, WI\"\t55123\n\"Juneau County, WI\"\t55057\t\"Wood County, WI\"\t55141\n\"Kenosha County, WI\"\t55059\t\"Lake County, IL\"\t17097\n\"Kenosha County, WI\"\t55059\t\"McHenry County, IL\"\t17111\n\"Kenosha County, WI\"\t55059\t\"Allegan County, MI\"\t26005\n\"Kenosha County, WI\"\t55059\t\"Kenosha County, WI\"\t55059\n\"Kenosha County, WI\"\t55059\t\"Racine County, WI\"\t55101\n\"Kenosha County, WI\"\t55059\t\"Walworth County, WI\"\t55127\n\"Kewaunee County, WI\"\t55061\t\"Benzie County, MI\"\t26019\n\"Kewaunee County, WI\"\t55061\t\"Manistee County, MI\"\t26101\n\"Kewaunee County, WI\"\t55061\t\"Brown County, WI\"\t55009\n\"Kewaunee County, WI\"\t55061\t\"Door County, WI\"\t55029\n\"Kewaunee County, WI\"\t55061\t\"Kewaunee County, WI\"\t55061\n\"Kewaunee County, WI\"\t55061\t\"Manitowoc County, WI\"\t55071\n\"La Crosse County, WI\"\t55063\t\"Houston County, MN\"\t27055\n\"La Crosse County, WI\"\t55063\t\"Winona County, MN\"\t27169\n\"La Crosse County, WI\"\t55063\t\"Jackson County, WI\"\t55053\n\"La Crosse County, WI\"\t55063\t\"La Crosse County, WI\"\t55063\n\"La Crosse County, WI\"\t55063\t\"Monroe County, WI\"\t55081\n\"La Crosse County, WI\"\t55063\t\"Trempealeau County, WI\"\t55121\n\"La Crosse County, WI\"\t55063\t\"Vernon County, WI\"\t55123\n\"Lafayette County, WI\"\t55065\t\"Jo Daviess County, IL\"\t17085\n\"Lafayette County, WI\"\t55065\t\"Stephenson County, IL\"\t17177\n\"Lafayette County, WI\"\t55065\t\"Grant County, WI\"\t55043\n\"Lafayette County, WI\"\t55065\t\"Green County, WI\"\t55045\n\"Lafayette County, WI\"\t55065\t\"Iowa County, WI\"\t55049\n\"Lafayette County, WI\"\t55065\t\"Lafayette County, WI\"\t55065\n\"Langlade County, WI\"\t55067\t\"Forest County, WI\"\t55041\n\"Langlade County, WI\"\t55067\t\"Langlade County, WI\"\t55067\n\"Langlade County, WI\"\t55067\t\"Lincoln County, WI\"\t55069\n\"Langlade County, WI\"\t55067\t\"Marathon County, WI\"\t55073\n\"Langlade County, WI\"\t55067\t\"Menominee County, WI\"\t55078\n\"Langlade County, WI\"\t55067\t\"Oconto County, WI\"\t55083\n\"Langlade County, WI\"\t55067\t\"Oneida County, WI\"\t55085\n\"Langlade County, WI\"\t55067\t\"Shawano County, WI\"\t55115\n\"Lincoln County, WI\"\t55069\t\"Langlade County, WI\"\t55067\n\"Lincoln County, WI\"\t55069\t\"Lincoln County, WI\"\t55069\n\"Lincoln County, WI\"\t55069\t\"Marathon County, WI\"\t55073\n\"Lincoln County, WI\"\t55069\t\"Oneida County, WI\"\t55085\n\"Lincoln County, WI\"\t55069\t\"Price County, WI\"\t55099\n\"Lincoln County, WI\"\t55069\t\"Taylor
